vi "Main.vi"() -> ()   [LabVIEW 2015]
doc: "Main method for the Colton Lab Scan Software. Entry point for a complied executable application."
uses:
  Global/Flags.vi
  Global/Misc.vi
  Scan Driver/Scan Driver.lvclass
panel:
  out "setVIdone":bool
  out "instrVIdone":bool
  # "Driver - Runs the \"Main\" Program"
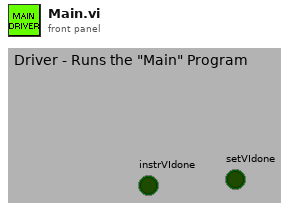
[diagram p1: front panel]
types:
  T1 = enum32{"Bad", "Idle", "Run top level", "Running"}
  T2 = enum32{"Invalid", "Standard", "Closed", "Hidden", "Minimized", "Maximized"}
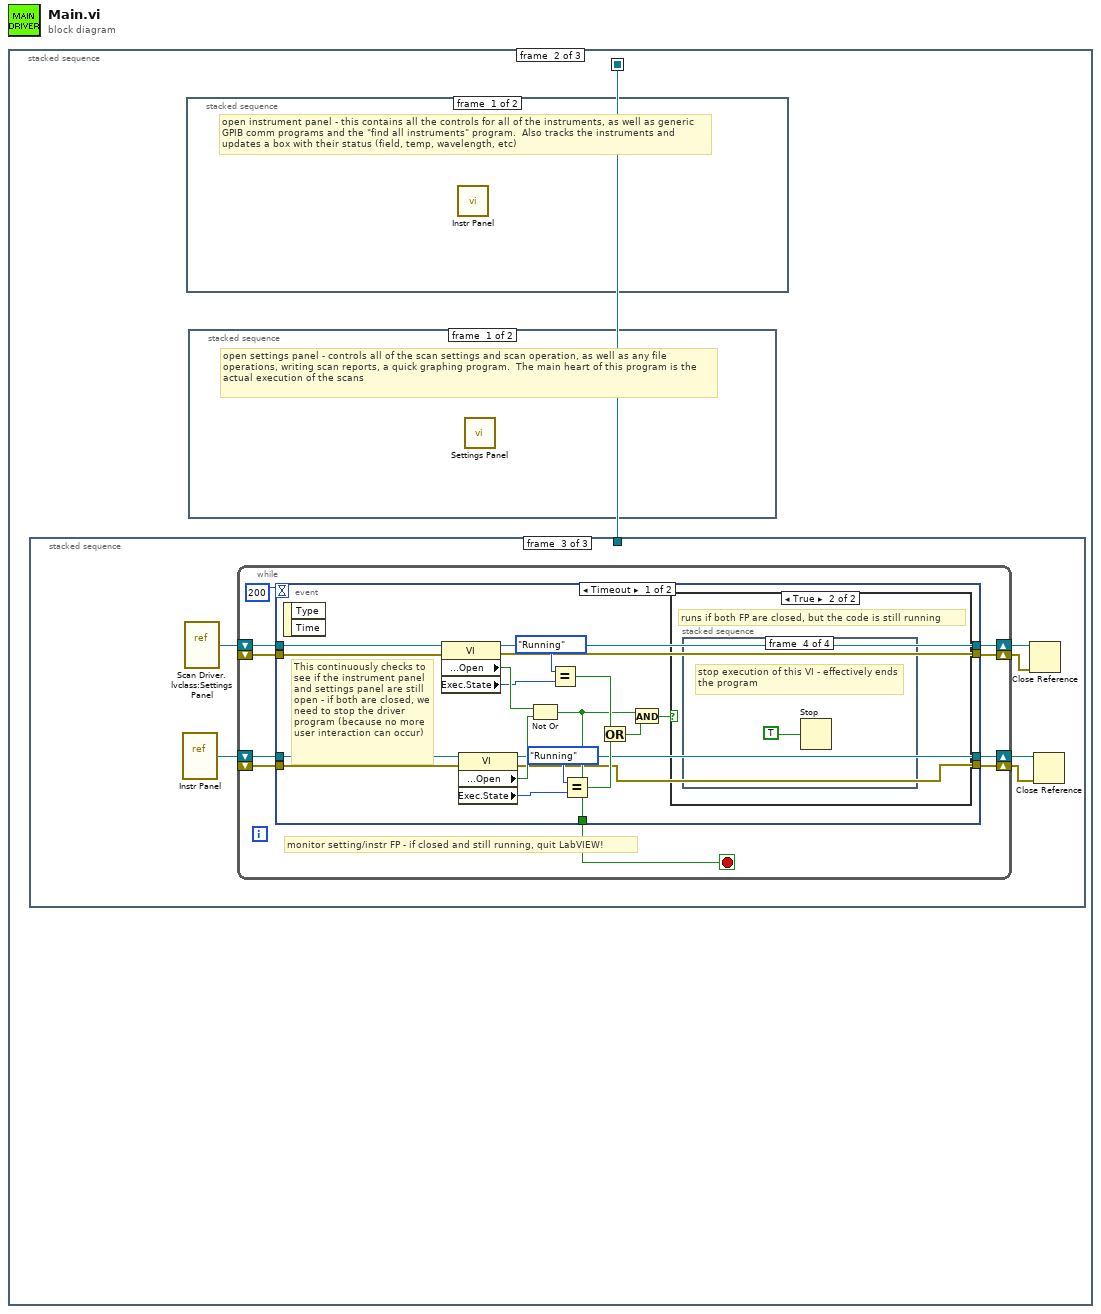
[diagram p0: block diagram]
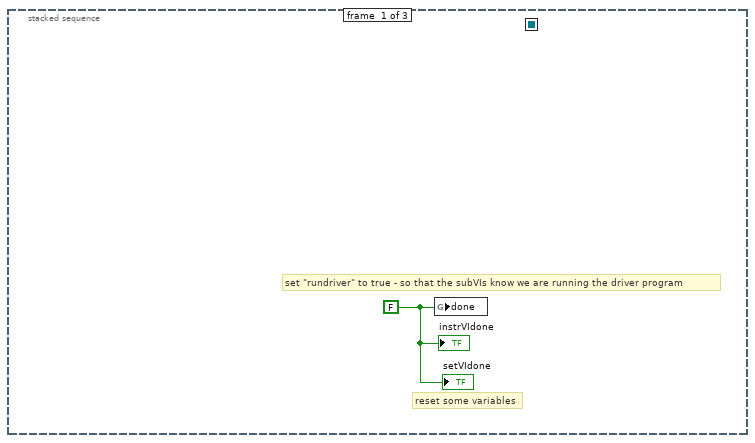
[diagram p2: hidden frame]
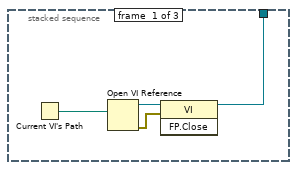
[diagram p3: hidden frame]
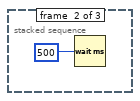
[diagram p4: hidden frame]
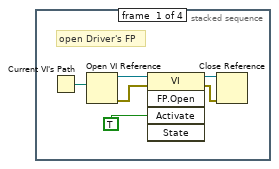
[diagram p6: hidden frame]
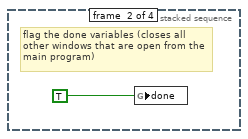
[diagram p7: hidden frame]
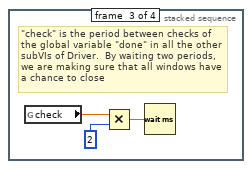
[diagram p8: hidden frame]
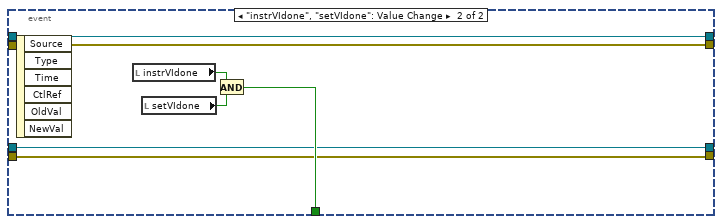
[diagram p9: hidden frame]
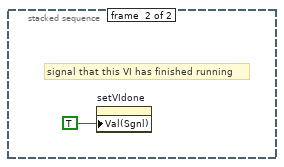
[diagram p10: hidden frame]
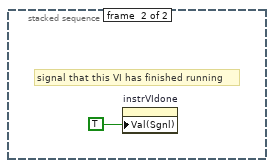
[diagram p11: hidden frame]
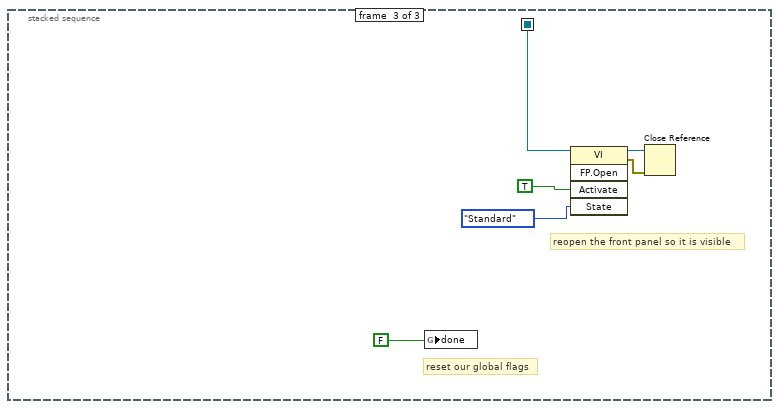
[diagram p12: hidden frame]
diagram:
  n1 = stacked-sequence {
    seq-local: [_ w2 _] -> [_ _ w68]
    frame #0 {
      w1 = FALSE
      # "reset some variables"
      # "set \"rundriver\" to true - so that the subVIs know we are running the driver program"
      n2 = global write "Flags.vi" "done"(w1) -> ()
      "instrVIdone" <- w1
      "setVIdone" <- w1
    }
    frame #1 {
      n3 = stacked-sequence {
        tunnel: [w5 _ _] -> w2
        frame #0 {
          n4 = Current VI's Path() -> (path=w4:path)
          n5 = Open VI Reference(vi path=w4) -> (vi reference=w6:refnum<vi>, error out=w3:errorcluster)  [unwired: 1 in, 4 out]
          n6 = invoke class="VI" method="FP.Close"(reference=w6, error in=w3) -> (reference out=w5:refnum<vi>)  [unwired: 1 in, 2 out]
        }
        frame #1 {
          n7 = Wait (ms)(milliseconds to wait=500) -> ()  [unwired: 1 out]
        }
        frame #2 {
          n8 = vi-ref "Instr Panel.vi"() -> (w9:refnum<vi>)
          n9 = vi-ref "Scan Driver.lvclass:Settings Panel.vi"() -> (w8:refnum<vi>)
          n10 = while {
            shift-right: [w18] -> w10
            shift-left: _ -> [w21]
            shift-right: [w19] -> w12
            shift-left: _ -> [w20]
            shift-right: [w15] -> w11
            shift-left: w8 -> [w17]
            shift-right: [w14] -> w13
            shift-left: w9 -> [w16]
            stop <- w22 stop-if-true
            # "monitor setting/instr FP - if closed and still running, quit LabVIEW!"
            n11 = event shown="[0] Timeout" {
              selector: _ -> [_ _]
              dyn-events: _ -> [_ _]
              timeout: 200 -> [_ _]
              tunnel: [w33 w58] -> w22
              tunnel: w21 -> [w28 w56]
              tunnel: w20 -> [w25 w54]
              tunnel: [w29 w54] -> w19
              tunnel: [w26 w56] -> w18
              tunnel: w17 -> [w31 w57]
              tunnel: w16 -> [w30 w55]
              tunnel: [w27 w57] -> w15
              tunnel: [w24 w55] -> w14
              event Timeout {
                # "This continuously checks to see if the instrument panel and settings panel are still open - if both are closed, we need to stop the driver program (because no more user interaction can occur)"
                n12 = event-data() -> ()  [unwired: 3 out]
                n13 = property class="VI"(reference=w31, error in=w28) -> (reference out=w27:refnum<vi>, error out=w26:errorcluster, "Front Panel.Open"=w42:bool, "Exec.State"=w39:T1)
                n14 = property class="VI"(reference=w30, error in=w25) -> (reference out=w24:refnum<vi>, error out=w29:errorcluster, "Front Panel.Open"=w41:bool, "Exec.State"=w37:T1)
                n15 = Not Or(1:w41, 2:w42) -> (0:w33:bool)
                n16 = Equal?(x=T1."Running" ("Execution:State"), y=w39) -> (x = y?=w36:bool)
                n17 = Equal?(x=T1."Running" ("Execution:State"), y=w37) -> (x = y?=w35:bool)
                n18 = Or(x=w36, y=w35) -> (x .or. y?=w34:bool)
                n19 = And(x=w33, y=w34) -> (x .and. y?=w32:bool)
                n20 = case shown="True" w32 {
                  frame False {
                  }
                  frame True {
                    # "runs if both FP are closed, but the code is still running"
                    n21 = stacked-sequence {
                      frame #0 {
                        # "open Driver's FP"
                        n22 = Current VI's Path() -> (path=w48:path)
                        n23 = Open VI Reference(vi path=w48) -> (vi reference=w47:refnum<vi>, error out=w46:errorcluster)  [unwired: 1 in, 4 out]
                        n24 = invoke class="VI" method="FP.Open"(reference=w47, error in=w46, "Activate"=TRUE) -> (reference out=w44:refnum<vi>, error out=w45:errorcluster)  [unwired: 2 in, 3 out]
                        n25 = Close Reference(reference=w44, error in (no error)=w45) -> ()  [unwired: 1 out]
                      }
                      frame #1 {
                        # "flag the done variables (closes all other windows that are open from the main program)"
                        n26 = global write "Flags.vi" "done"(TRUE) -> ()
                      }
                      frame #2 {
                        # "\"check\" is the period between checks of the global variable \"done\" in all the other subVIs of Driver.  By waiting two periods, we are making sure that all windows have a chance to close"
                        n27 = global read "Misc.vi" "check"() -> (w52:dbl)
                        n28 = Multiply(x=w52, y=2) -> (x*y=w50:dbl)
                        n29 = Wait (ms)(milliseconds to wait=w50) -> ()  [unwired: 1 out]
                      }
                      frame #3 {
                        # "stop execution of this VI - effectively ends the program"
                        n30 = Stop(stop? (T)=TRUE) -> ()
                      }
                    }
                  }
                }
              }
              event "instrVIdone", "setVIdone": Value Change {
                n31 = event-data() -> ()  [unwired: 7 out]
                n32 = local read "instrVIdone"() -> (w60:bool)
                n33 = local read "setVIdone"() -> (w59:bool)
                n34 = And(x=w60, y=w59) -> (x .and. y?=w58:bool)
              }
            }
          }
          n35 = Close Reference(reference=w11, error in (no error)=w10) -> ()  [unwired: 1 out]
          n36 = Close Reference(reference=w13, error in (no error)=w12) -> ()  [unwired: 1 out]
        }
      }
      n37 = stacked-sequence {
        frame #0 {
          # "open instrument panel - this contains all the controls for all of the instruments, as well as generic GPIB comm programs and the \"find all instruments\" program.  Also tracks the instruments and updates a box with their status (field, temp, wavelength, etc)"
          n38 = call "Instr Panel.vi"() -> ()  [unwired: 1 out]
        }
        frame #1 {
          # "signal that this VI has finished running"
          n39 = property on="instrVIdone" class="Bool (strict)"("Val(Sgnl)"=TRUE) -> ()  [unwired: 2 in, 2 out]
        }
      }
      n40 = stacked-sequence {
        frame #0 {
          # "open settings panel - controls all of the scan settings and scan operation, as well as any file operations, writing scan reports, a quick graphing program.  The main heart of this program is the actual execution of the scans"
          n41 = call "Settings Panel.vi"() -> ()  [unwired: 1 out]
        }
        frame #1 {
          # "signal that this VI has finished running"
          n42 = property on="setVIdone" class="Bool (strict)"("Val(Sgnl)"=TRUE) -> ()  [unwired: 2 in, 2 out]
        }
      }
    }
    frame #2 {
      # "reset our global flags"
      # "reopen the front panel so it is visible"
      n43 = global write "Flags.vi" "done"(FALSE) -> ()
      n44 = invoke class="VI" method="FP.Open"(reference=w68, "Activate"=TRUE, "State"=T2."Standard") -> (reference out=w64:refnum<vi>, error out=w63:errorcluster)  [unwired: 2 in, 3 out]
      n45 = Close Reference(reference=w64, error in (no error)=w63) -> ()  [unwired: 1 out]
    }
  }
